vi "Read Binary.vi"(6 "error in (no error)":errorcluster, 8 "timeout ms (5000)":i32=5000, 9 "ICommHandler in":refnum<class "ICommHandler.lvclass">) -> (0 "error out":errorcluster, 1 "Bytes":u8[](array[numeric]), 3 "ICommHandler out":refnum<class "ICommHandler.lvclass">)   [LabVIEW 2020, in "wamplv.lvlib" / "ICommHandler.lvclass"]
uses:
  ICommHandler.lvclass
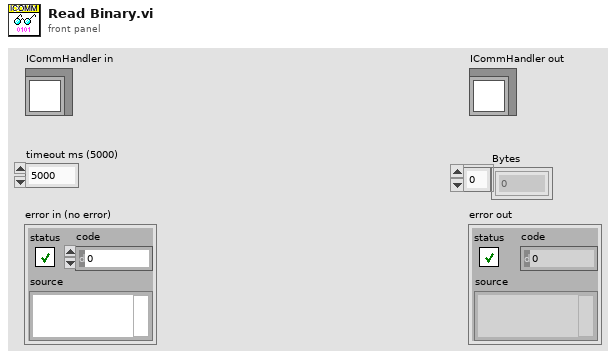
[diagram p1: front panel]
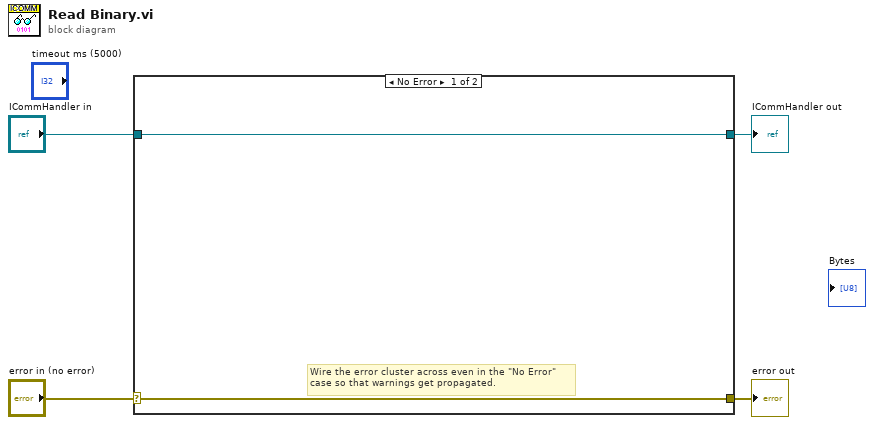
[diagram p0: block diagram]
diagram:
  n1 = case shown="No Error" "error in (no error)" {
    selector: "error in (no error)" -> [w5 w8]
    tunnel: [w5 w8] -> w3
    tunnel: [w6 w7] -> w1
    tunnel: "ICommHandler in" -> [w6 w7]
    frame No Error {
      # "Wire the error cluster across even in the \"No Error\"\ncase so that warnings get propagated."
    }
    frame Error {
    }
  }
  "error out" <- w3
  "ICommHandler out" <- w1
